vi "Andor_Operate.vi"(8 "error in (no error)":errorcluster, 10 "AndorMainQ":refnum<queue>, 11 "AndorOpQ":refnum<queue>) -> (0 "error out":errorcluster)   [LabVIEW 2019]
uses:
  <userlib>/ATSpectrograph/GUI/AndorNoiseCorr.ctl
  <vilib>/Utility/error.llb/DialogType.ctl
  <userlib>/atmcd32d.llb/Error Code Enum typedef.ctl
panel:
  out "avgfac":i32
  out "Thresh":sgl
  out "cosmic filter":bool
  in  "FilterMode":u32
  out "Dll Error Code":u32
  in  "test filter":bool
  in  "#Curves":u32=1 min=1 max=20 step=1
  out "TempErr":bool
  in  "Backgnd Mode":T1
  out "Background":i32[](array[numeric])
  in  "Standalone":bool
  out "Temp °C":i32
  out "Stable":bool
  in  "Setp. °C":i32=-80
  in  "Quit":bool
  out "CalValues":sgl[](array[numeric])
  in  "Gain":i32(ring) caption="Device Name" items=["Gain  1.0(x)", "Gain  1.7(x)"]
  out "Aquiring":bool
  in  "Continuous Acq.":bool
  in  "AcquireImage":bool
  out "Datas":i32[][][](array[numeric])
  out "Acq Time(ms)":u32
  in  "Accumulations":u16=1 min=1 step=1
  in  "Cooler Enable":bool=TRUE
  in  "Int_time(ms)":u32=10 caption="Integration time(ms)"
  out "Connected":bool
  in  "Stop":bool
  in  "Init":bool
  in  "Tab Control":enum32{"Spectre", "Image"}(tab)
  out "Max WL":sgl
  out "Sum":dbl
  out "Max":u32
  out "Delta":i32
  out "Max X Position":i32[](array[numeric])
  out "Spectral Graph":cluster{"CalValues":sgl[], dbl[]}[](graph)
  out "Max Intensity":i32[](array[numeric])
  out "Graph":dbl[][](graph)
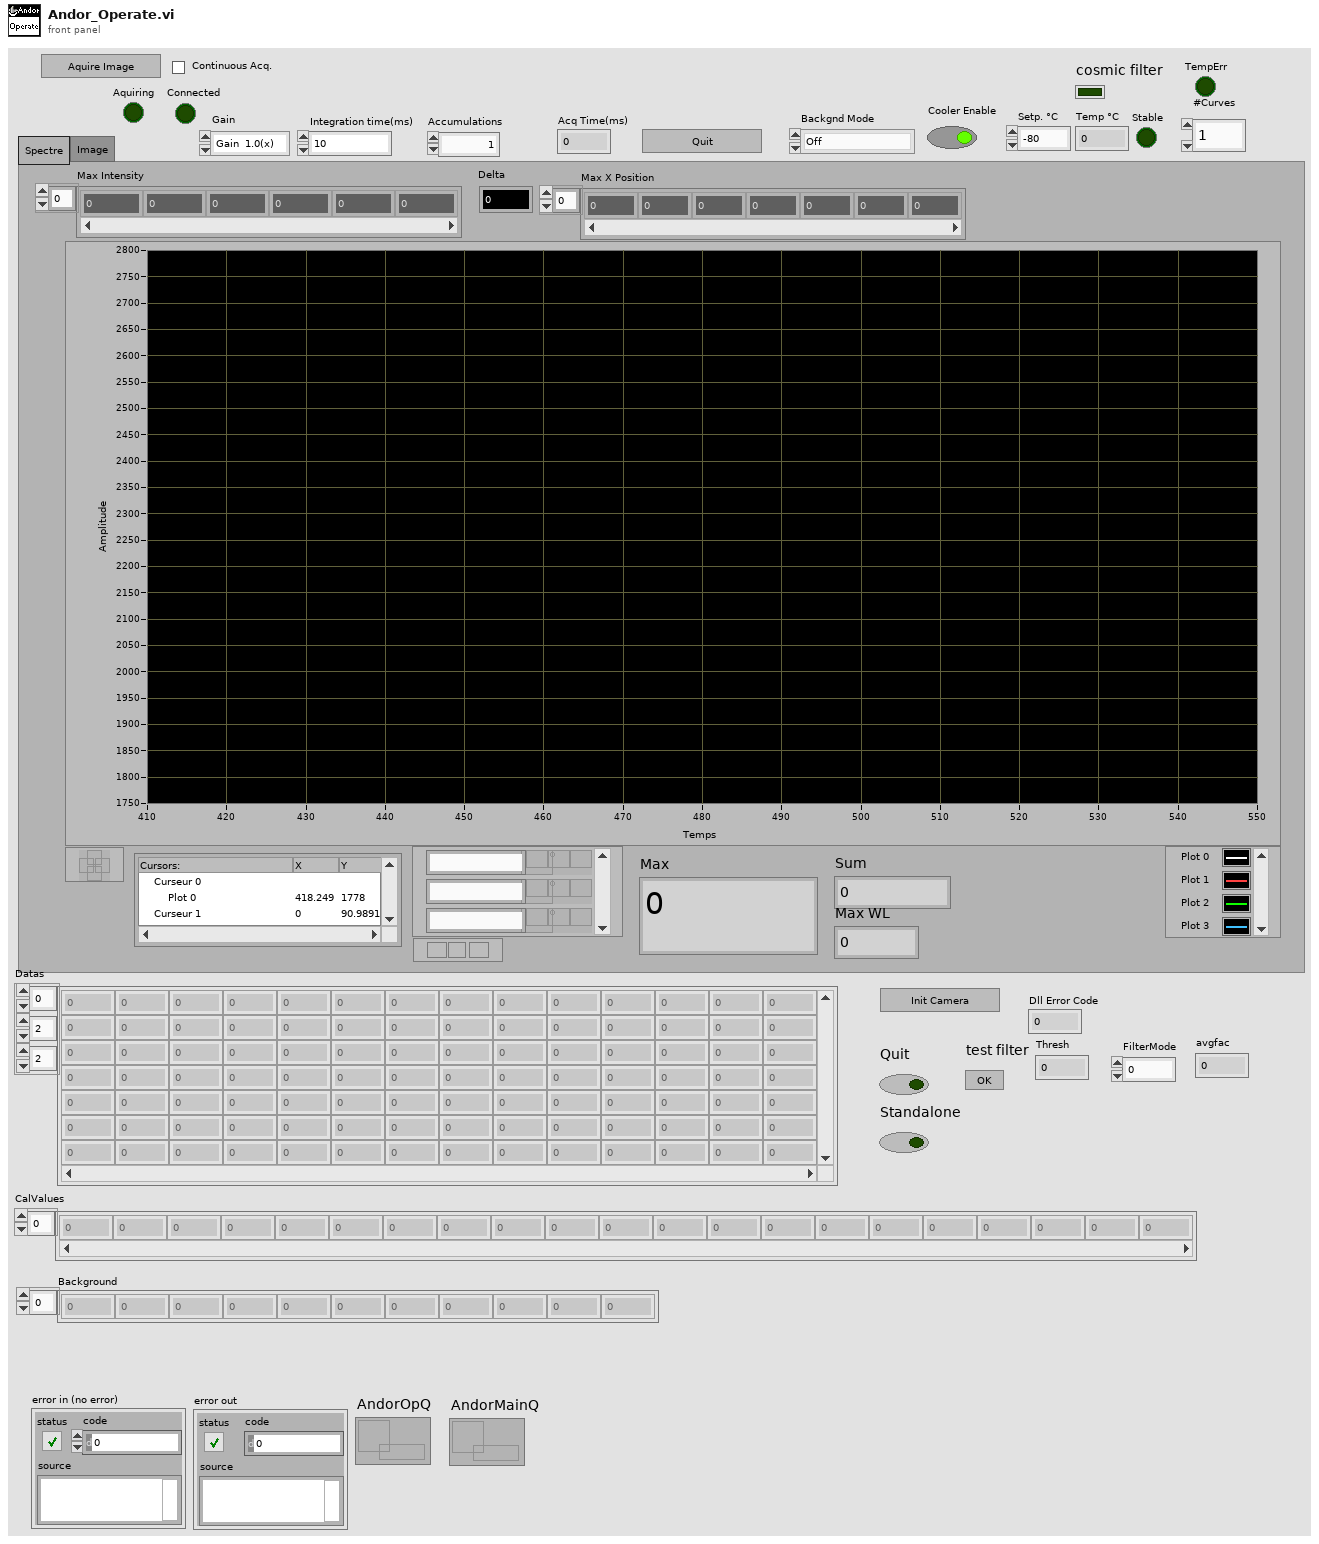
[diagram p1: front panel]
types:
  T1 = typedef "AndorNoiseCorr.ctl" = enum16{"Off", "Selected Curve", "One For Every Acq"}
  T2 = typedef "Error Code Enum typedef.ctl" = enum32{"N/A (0)", "DRV_ERROR_CODES", "DRV_SUCCESS", "DRV_VXDNOTINSTALLED", "DRV_ERROR_SCAN", "DRV_ERROR_CHECK_SUM", "DRV_ERROR_FILELOAD", "DRV_UNKNOWN_FUNC", "DRV_ERROR_VXD_INIT", "DRV_ERROR_ADDRESS", "DRV_ERROR_PAGELOCK", "DRV_ERROR_PAGEUNLOCK", "DRV_ERROR_BOARDTEST", "DRV_ERROR_ACK", "DRV_ERROR_UP_FIFO", "DRV_ERROR_PATTERN", "N/A (16)", "DRV_ACQUISITION_ERRORS", "DRV_ACQ_BUFFER", "DRV_ACQ_DOWNFIFO_FULL", "DRV_PROC_UNKONWN_INSTRUCTION", "DRV_ILLEGAL_OP_CODE", "DRV_KINETIC_TIME_NOT_MET", "DRV_ACCUM_TIME_NOT_MET", "DRV_NO_NEW_DATA", "N/A (25)", "DRV_SPOOLERROR", "N/A (27)", "N/A (28)", "N/A (29)", "N/A (30)", "N/A (31)", "N/A (32)", "DRV_TEMPERATURE_CODES", "DRV_TEMPERATURE_OFF", "DRV_TEMPERATURE_NOT_STABILIZED", "DRV_TEMPERATURE_STABILIZED", "DRV_TEMPERATURE_NOT_REACHED", "DRV_TEMPERATURE_OUT_RANGE", "DRV_TEMPERATURE_NOT_SUPPORTED", "DRV_TEMPERATURE_DRIFT", "N/A (41)", "N/A (42)", "N/A (43)", "N/A (44)", "N/A (45)", "N/A (46)", "N/A (47)", "N/A (48)", "DRV_GENERAL_ERRORS", "DRV_INVALID_AUX", "DRV_COF_NOTLOADED", "DRV_FPGAPROG", "DRV_FLEXERROR", "DRV_GPIBERROR", "N/A (55)", "N/A (56)", "N/A (57)", "N/A (58)", "N/A (59)", "N/A (60)", "N/A (61)", "N/A (62)", "N/A (63)", "DRV_DATATYPE", "DRV_DRIVER_ERRORS", "DRV_P1INVALID", "DRV_P2INVALID", "DRV_P3INVALID", "DRV_P4INVALID", "DRV_INIERROR", "DRV_COFERROR", "DRV_ACQUIRING", "DRV_IDLE", "DRV_TEMPCYCLE", "DRV_NOT_INITIALIZED", "DRV_P5INVALID", "DRV_P6INVALID", "DRV_INVALID_MODE", "DRV_INVALID_FILTER", "DRV_I2CERRORS", "DRV_I2CDEVNOTFOUND", "DRV_I2CTIMEOUT", "DRV_P7INVALID", "N/A (84)", "N/A (85)", "N/A (86)", "N/A (87)", "N/A (88)", "N/A (89)", "DRV_IOCERROR", "DRV_VRMVERSIONERROR"}
  T3 = cluster{"Message":string, "Data":variant, "Code":i32}
  T4 = cluster{"wavelength out":sgl, "calibrationValuesOut":sgl[], "gain":sgl, bool}
  T5 = typedef "DialogType.ctl" = u16
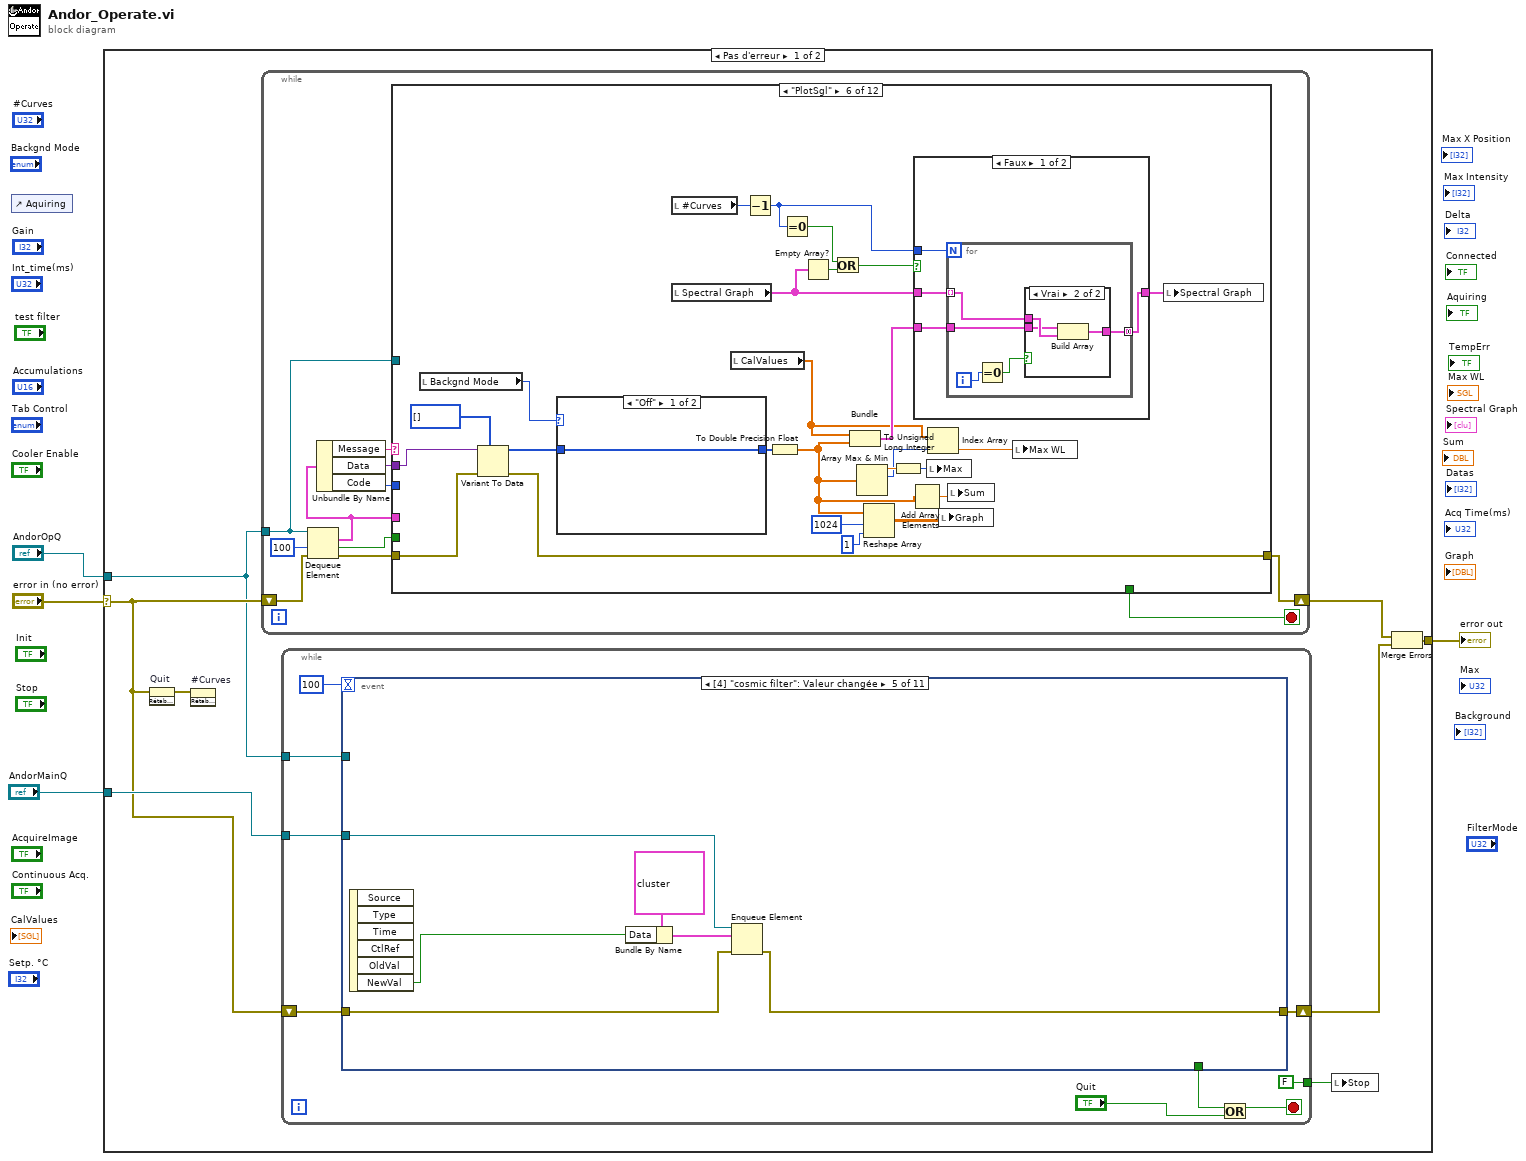
[diagram p0: block diagram]
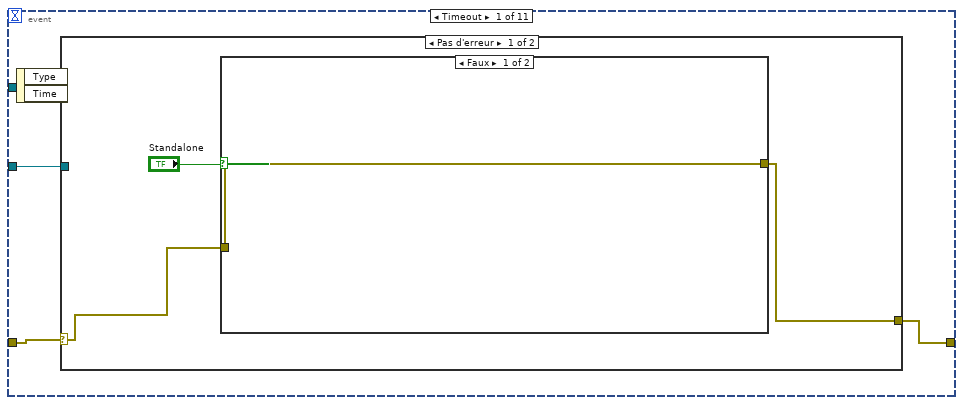
[diagram p2: hidden frame]
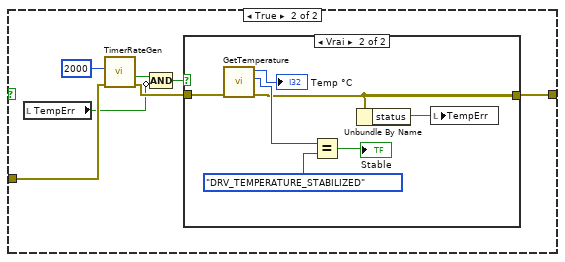
[diagram p3: hidden frame]
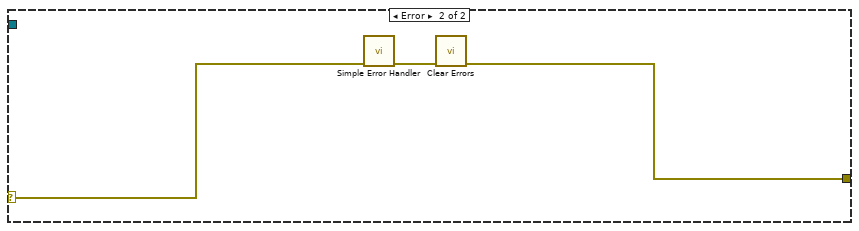
[diagram p5: hidden frame]
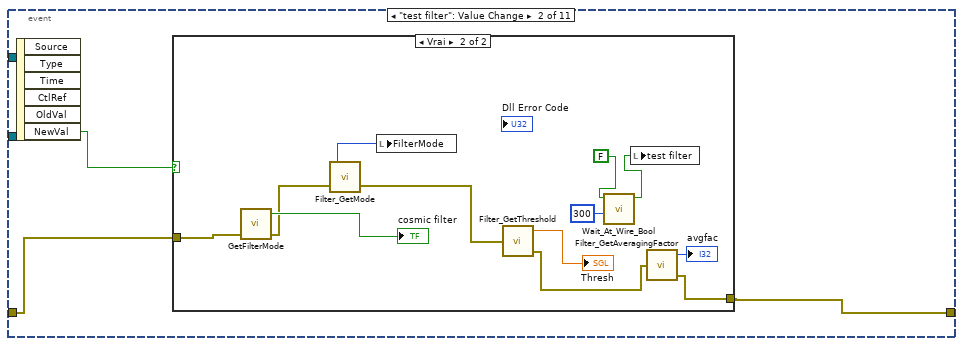
[diagram p6: hidden frame]
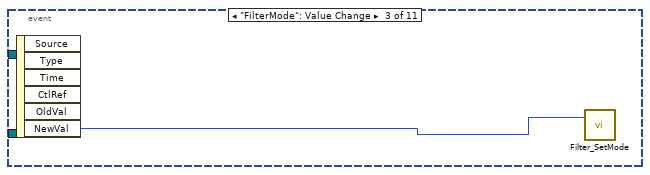
[diagram p8: hidden frame]
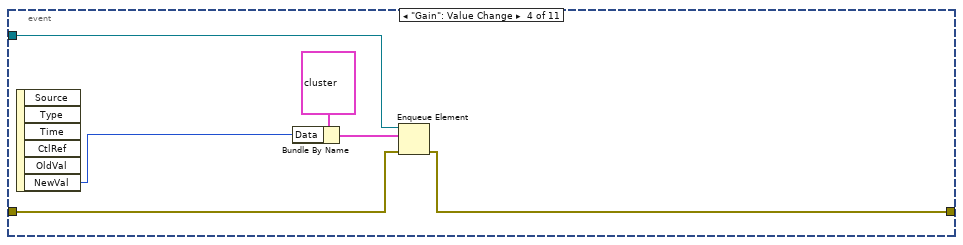
[diagram p9: hidden frame]
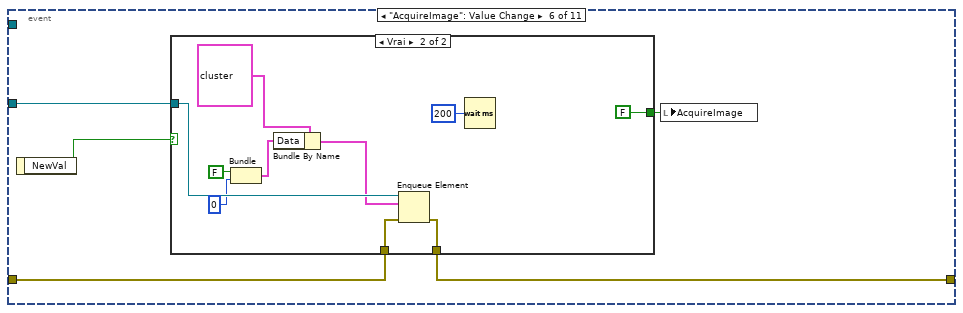
[diagram p10: hidden frame]
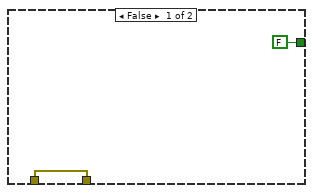
[diagram p11: hidden frame]
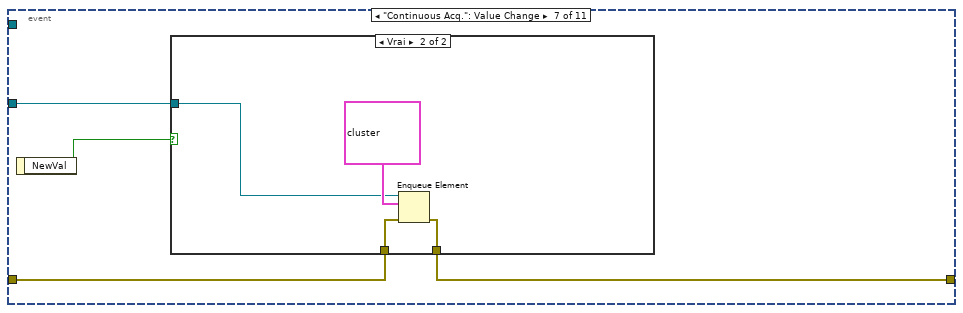
[diagram p12: hidden frame]
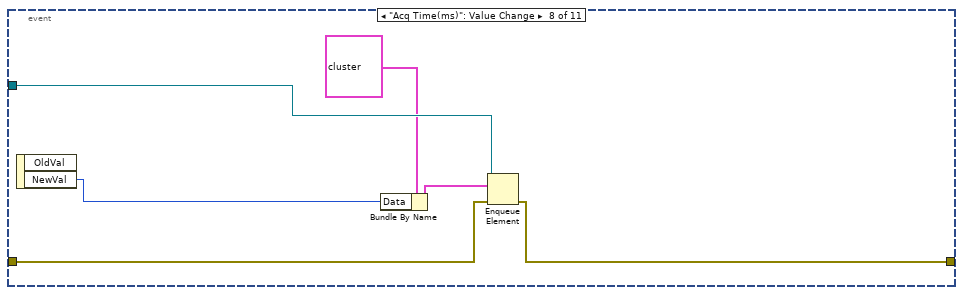
[diagram p14: hidden frame]
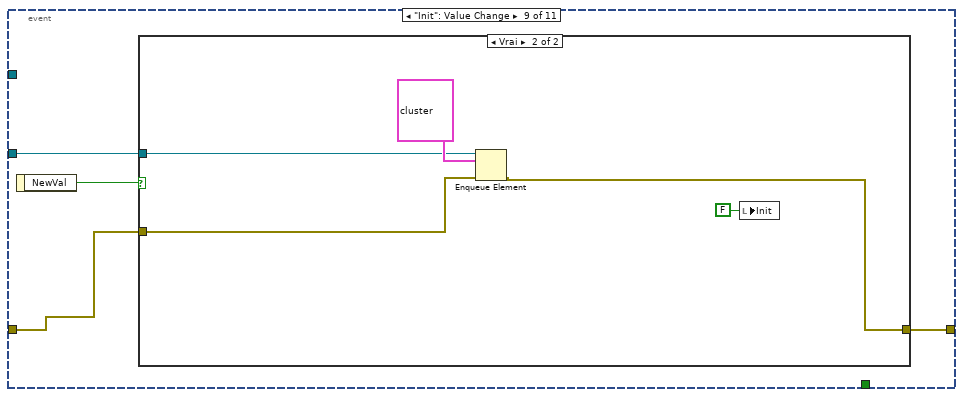
[diagram p15: hidden frame]
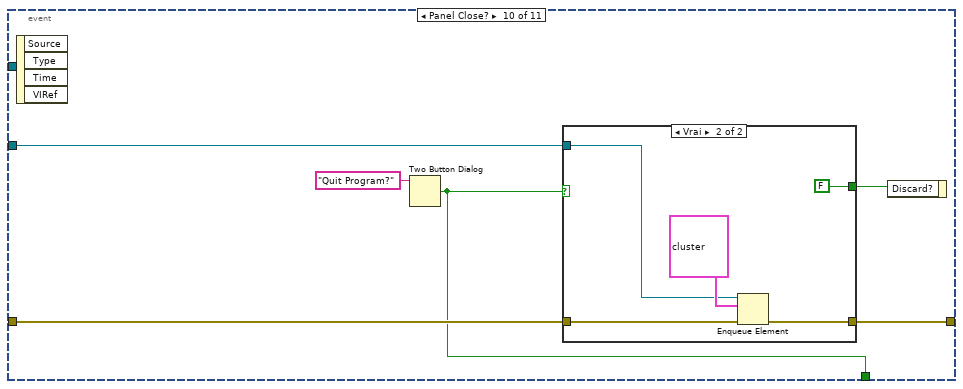
[diagram p17: hidden frame]
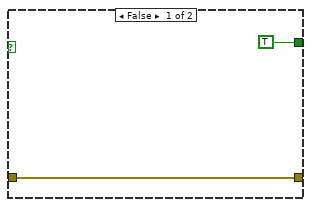
[diagram p18: hidden frame]
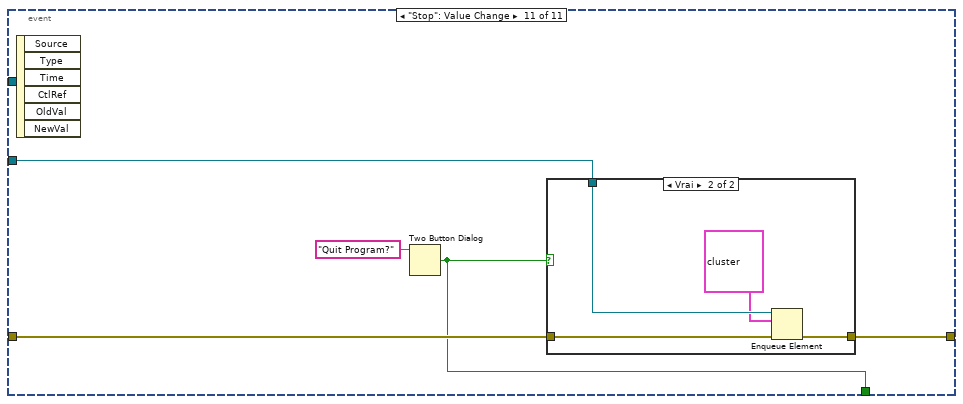
[diagram p19: hidden frame]
diagram:
  n1 = control-ref of="Aquiring"() -> ()  [unwired: 1 out]
  n2 = case shown="Pas d'erreur" "error in (no error)" {
    selector: "error in (no error)" -> [w8 w287]
    tunnel: [w12 w287] -> w3
    tunnel: "AndorMainQ" -> [w10 _]
    tunnel: "AndorOpQ" -> [w7 _]
    frame No Error {
      n3 = invoke on="Quit" class="Bool (strict)" method="RétablirValParDéfaut"(error in=w8) -> (error out=w5:errorcluster)  [unwired: 2 in, 2 out]
      n4 = invoke on="#Curves" class="NumNb (strict)" method="RétablirValParDéfaut"(error in=w5) -> ()  [unwired: 2 in, 3 out]
      n5 = while {
        shift-right: [w141] -> w9
        shift-left: w8 -> [w151]
        tunnel: w7 -> [w145]
        stop <- w148 stop-if-true
        n6 = Dequeue Element(queue=w145, timeout in ms (-1)=100, error in (no error)=w151) -> (element=w146:T3, timed out?=w142:bool, error out=w150:errorcluster)  [unwired: 1 out]
        n7 = Unbundle By Name(w146) -> ("Message"=w149:string, "Data"=w143:variant, "Code"=w144:i32)
        n8 = case shown="\"PlotSgl\"" w149 {
          tunnel: [w152 w158 w164 w191 w196 w223 w254 w262 w268 w274 w279 w284] -> w141
          tunnel: w150 -> [w154 w159 w163 w180 w199 w224 w255 w263 w269 w275 w280 w285]
          tunnel: [w156 FALSE w162 FALSE FALSE _ _ _ _ _ _ _] -> w148
          tunnel: w146 -> [_ _ _ _ _ _ _ _ _ _ _ _]
          tunnel: w145 -> [w155 w160 _ _ _ _ _ _ _ _ _ _]
          tunnel: w144 -> [_ _ _ _ _ _ _ _ _ _ _ _]
          tunnel: w143 -> [_ _ _ w185 w200 w226 w257 w266 w271 w276 w281 w286]
          tunnel: w142 -> [_ _ _ _ _ _ _ _ _ _ _ _]
          frame "Stop" {
            w156 = TRUE
            n9 = Release Queue(queue=w155, error in (no error)=w154) -> (error out=w153:errorcluster)  [unwired: 1 in, 2 out]
            n10 = property on="Quit" class="Bool (strict)"(error in=w153, "Val(Sgnl)"=w156) -> (error out=w152:errorcluster)  [unwired: 1 in, 1 out]
          }
          frame "Standalone" {
            n11 = local write "Standalone"(TRUE ("Standalone")) -> ()
            n12 = Release Queue(queue=w160, error in (no error)=w159) -> (error out=w158:errorcluster)  [unwired: 1 in, 2 out]
          }
          frame "Timeout", Default {
            n13 = Unbundle By Name(w163) -> ("code"=w166:i32)
            n14 = Equal?(x=w166, y=1) -> (x = y?=w162:bool)
            n15 = case shown="Faux" w162 {
              tunnel: [w168 w171] -> w164
              tunnel: w163 -> [w167 w171]
              frame False {
                w170 = T5 1 items=["pas de dialogue", "Message OK", "Message continuer ou arrêter", "Message OK + mises en garde", "Arrêter/Continuer + mises en garde"] ("type of dialog (OK msg:1)")
                n16 = call <vilib>:"General Error Handler.vi"("type of dialog (OK msg:1)"=w170, "error in (no error)"=w167) -> ("error out"=w169:errorcluster)  [unwired: 9 in, 4 out]
                n17 = local write "error out"(w169) -> ()
                n18 = call <vilib>:"Clear Errors.vi"("error in (no error)"=w169) -> ("error out"=w168:errorcluster)  [unwired: 5 in, 1 out]
              }
              frame True {
              }
            }
          }
          frame "InitOp" {
            n19 = invoke on="Connected" class="Bool (strict)" method="RétablirValParDéfaut"(error in=w180) -> (error out=w187:errorcluster)  [unwired: 2 in, 2 out]
            n20 = Reverse 1D Array(array=u32[] [16711680, 16773120, 2359040, 131327, 3080307] ("Sous-tableau")) -> (reversed array=w189:u32[])
            n21 = Variant To Data(error in=w180, type=T4 {"wavelength out"=0.0, "calibrationValuesOut"=[], "gain"=0.0, FALSE} ("cluster"), Variant=w185) -> (data=w183:T4, error out=w182:errorcluster)
            n22 = for {
              tunnel: cluster{dbl, u32}[] [{0.0, 0}, {10923.0, 0}, {21845.0, 0}, {32768.0, 0}, {43691.0, 0}, {54613.0, 0}] ("Z Scale.Marker Values[]") -> [w195] mode=indexing
              tunnel: w189 -> [w194] mode=indexing
              tunnel: [w193] -> w181 mode=indexing
              n23 = Bundle(cluster=w195, w194) -> (w193:cluster{dbl, u32})  [unwired: 1 in]
            }
            n24 = Unbundle By Name(w183) -> ("calibrationValuesOut"=w186:sgl[])  [unwired: 2 out]
            n25 = invoke on="Accumulations" class="NumNb (strict)" method="RétablirValParDéfaut"(error in=w187) -> (error out=w178:errorcluster)  [unwired: 2 in, 2 out]
            n26 = invoke on="Standalone" class="Bool (strict)" method="RétablirValParDéfaut"(error in=w178) -> (error out=w177:errorcluster)  [unwired: 2 in, 2 out]
            n27 = Initialize Array(0, 1024 ("taille de la dimension")) -> (w175:i32[])
            n28 = property on="Graph" class="GraphInt (strict)"(error in=w180, "ZScale.MarkerVals[]"=w181) -> (error out=w179:errorcluster)  [unwired: 1 in, 1 out]
            n29 = local write "CalValues"(w186) -> ()
            n30 = local write "Background"(w175) -> ()
            n31 = invoke on="Backgnd Mode" class="Énum (strict)" method="RétablirValParDéfaut"(error in=w177) -> (error out=w176:errorcluster)  [unwired: 2 in, 2 out]
            n32 = local write "TempErr"(FALSE ("TempErr")) -> ()
            n33 = Merge Errors(w176, w182, w179) -> (w191:errorcluster)
          }
          frame "UpdateWl" {
            n34 = Variant To Data(error in=w199, type=sgl[] [] ("calibrationValuesOut"), Variant=w200) -> (data=w197:sgl[], error out=w196:errorcluster)
            n35 = local write "CalValues"(w197) -> ()
          }
          frame "PlotSgl" {
            n36 = local read "Backgnd Mode"() -> (w217:T1)
            n37 = Variant To Data(error in=w224, type=i32[] [] ("Data out"), Variant=w226) -> (data=w215:i32[], error out=w223:errorcluster)
            n38 = case shown="\"Off\"" w217 {
              tunnel: [w243 w244] -> w216
              tunnel: w215 -> [w243 w246]
              frame "Off" {
              }
              frame "Selected Curve", Default {
                n39 = local read "Background"() -> (w245:i32[])
                n40 = Subtract(x=w246, y=w245) -> (x-y=w244:i32[])
              }
            }
            n41 = local read "#Curves"() -> (w211:u32)
            n42 = local read "Spectral Graph"() -> (w209:cluster{"CalValues":sgl[], dbl[]}[])
            n43 = local read "CalValues"() -> (w203:sgl[])
            n44 = Decrement(x=w211) -> (x-1=w210:u32)
            n45 = To Double Precision Float(number=w216) -> (double precision float=w206:dbl[])
            n46 = Equal To 0?(x=w210) -> (x = 0?=w212:bool)
            n47 = Empty Array?(array=w209) -> (empty?=w213:bool)
            n48 = Or(x=w212, y=w213) -> (x .or. y?=w208:bool)
            n49 = Bundle("CalValues"=w203, w206) -> (w214:cluster{"CalValues":sgl[], dbl[]})  [unwired: 1 in]
            n50 = Array Max & Min(array=w206) -> (max value=w219:dbl, max index (indices)=w204:i32)  [unwired: 2 out]
            n51 = Reshape Array(w206, 1024 ("taille de la dimension"), 1 ("taille de la dimension")) -> (w222:dbl[][])
            n52 = To Unsigned Long Integer(number=w219) -> (unsigned 32bit integer=w218:u32)
            n53 = Add Array Elements(numeric array=w206) -> (sum=w205:dbl)
            n54 = case shown="Faux" w208 {
              tunnel: w214 -> [w230 w242]
              tunnel: w210 -> [w229 _]
              tunnel: w209 -> [w228 _]
              tunnel: [w227 w241] -> w207
              frame False {
                n55 = for {
                  N: w229 -> [_]
                  tunnel: w228 -> [w233] mode=indexing
                  tunnel: w230 -> [w232]
                  tunnel: [w231] -> w227 mode=concatenating
                  i -> [w235]
                  n56 = Equal To 0?(x=w235) -> (x = 0?=w234:bool)
                  n57 = case shown="Vrai" w234 {
                    tunnel: w233 -> [w237 w240]
                    tunnel: w232 -> [_ w239]
                    tunnel: [w236 w238] -> w231
                    frame False {
                      n58 = Build Array(w237) -> (w236:cluster{"CalValues":sgl[], dbl[]}[])
                    }
                    frame True {
                      n59 = Build Array(w239, w240) -> (w238:cluster{"CalValues":sgl[], dbl[]}[])
                    }
                  }
                }
              }
              frame True {
                n60 = Build Array(w242) -> (w241:cluster{"CalValues":sgl[], dbl[]}[])
              }
            }
            n61 = local write "Max"(w218) -> ()
            n62 = Index Array(array=w203, index=w204) -> (element=w202:sgl)
            n63 = local write "Graph"(w222) -> ()
            n64 = local write "Sum"(w205) -> ()
            n65 = local write "Max WL"(w202) -> ()
            n66 = local write "Spectral Graph"(w207) -> ()
          }
          frame "PlotImg" {
            n67 = Variant To Data(error in=w255, type=i32[][] [] ("Data out"), Variant=w257) -> (data=w253:i32[][], error out=w254:errorcluster)
            n68 = local read "CalValues"() -> (w252:sgl[])
            n69 = To Double Precision Float(number=w253) -> (double precision float=w250:dbl[][])
            n70 = Transpose 2D Array(2D array=w250) -> (transposed array=w247:dbl[][])
            n71 = Array Max & Min(array=w247) -> (max value=w249:dbl)  [unwired: 3 out]
            n72 = for {
              tunnel: w250 -> [w260] mode=indexing
              tunnel: w252 -> [w259]
              tunnel: [w258] -> w251 mode=indexing
              n73 = Bundle("CalValues"=w259, w260) -> (w258:cluster{"CalValues":sgl[], dbl[]})  [unwired: 1 in]
            }
            n74 = local write "Graph"(w247) -> ()
            n75 = To Unsigned Long Integer(number=w249) -> (unsigned 32bit integer=w248:u32)
            n76 = local write "Max"(w248) -> ()
            n77 = local write "Spectral Graph"(w251) -> ()
          }
          frame "SetBckGnd" {
            n78 = Variant To Data(error in=w263, type=i32[][] [], Variant=w266) -> (data=w264:i32[][], error out=w262:errorcluster)
            n79 = Index Array(array=w264) -> (element=w261:i32[])  [unwired: 2 in]
            n80 = local write "Background"(w261) -> ()
          }
          frame "SetBckGndMode" {
            n81 = Variant To Data(error in=w269, type=u16 0, Variant=w271) -> (data=w270:u16, error out=w268:errorcluster)
            n82 = local write "Backgnd Mode"(w270) -> ()
          }
          frame "SetInteg" {
            n83 = Variant To Data(error in=w275, type=u32 0, Variant=w276) -> (data=w273:u32, error out=w274:errorcluster)
            n84 = local write "Int_time(ms)"(w273) -> ()
          }
          frame "SetCosmic" {
            n85 = Variant To Data(error in=w280, type=TRUE, Variant=w281) -> (data=w278:bool, error out=w279:errorcluster)
            n86 = local write "cosmic filter"(w278) -> ()
          }
          frame "SetGain" {
            n87 = Variant To Data(error in=w285, type=0, Variant=w286) -> (data=w283:i32, error out=w284:errorcluster)
            n88 = local write "Gain"(w283) -> ()
          }
        }
      }
      n89 = while {
        tunnel: w10 -> [w20]
        shift-right: [w17] -> w11
        shift-left: w8 -> [w18]
        tunnel: w7 -> [w14]
        tunnel: [FALSE ("Stop")] -> w6
        stop <- w16 stop-if-true
        n90 = event shown="[4] \"cosmic filter\": Valeur changée" {
          selector: _ -> [_ _ _ _ _ _ _ _ _ _ _]
          dyn-events: _ -> [_ _ _ _ _ _ _ _ _ _ _]
          timeout: 100 -> [_ _ _ _ _ _ _ _ _ _ _]
          tunnel: w20 -> [w22 _ _ w68 w74 w80 w96 w107 w110 w122 w134]
          tunnel: [_ _ _ _ _ _ _ _ _ w119 w131] -> w19
          tunnel: w18 -> [w23 w48 _ w67 w73 w79 w95 w106 w109 w121 w133]
          tunnel: [w24 w47 _ w66 w72 w78 w94 w105 w108 w120 w132] -> w17
          tunnel: w14 -> [_ _ _ _ _ _ _ _ _ _ _]
          event Timeout {
            n91 = event-data() -> ()  [unwired: 1 in, 2 out]
            n92 = case shown="Pas d'erreur" w23 {
              selector: w23 -> [w26 w44]
              tunnel: [w25 w45] -> w24
              tunnel: w22 -> [_ _]
              frame No Error {
                n93 = case shown="Faux" "Standalone" {
                  tunnel: w26 -> [w28 w34]
                  tunnel: [w28 w31] -> w25
                  frame False {
                  }
                  frame True {
                    n94 = local read "TempErr"() -> (w29:bool)
                    n95 = call <userlib>:"TimerRateGen.vi"("error in (no error)"=w34, "Refresh(ms)"=u32 2000) -> ("error out"=w33:errorcluster, "updated?"=w32:bool)  [unwired: 7 in, 1 out]
                    n96 = Compound Arithmetic op=AND ("Opérateur arithmétique")(w32, invert w29) -> (w30:bool)
                    n97 = case shown="Vrai" w30 {
                      tunnel: w33 -> [w36 w43]
                      tunnel: [w36 w38] -> w31
                      frame False {
                      }
                      frame True {
                        n98 = call <userlib>:"GetTemperature.vi"("error in (no error)"=w43) -> ("error out"=w38:errorcluster, "status"=w40:T2, "temperature"=→"Temp °C":i32)  [unwired: 3 in, 1 out]
                        n99 = Equal?(x=w40, y=Error_Code_Enum_typedef."DRV_TEMPERATURE_STABILIZED" ("status")) -> (x = y?=→"Stable":bool)
                        n100 = Unbundle By Name(w38) -> ("status"=w37:bool)
                        n101 = local write "TempErr"(w37) -> ()
                      }
                    }
                  }
                }
              }
              frame Error {
                n102 = call <vilib>:"Simple Error Handler.vi"("error in (no error)"=w44) -> ("error out"=w46:errorcluster)  [unwired: 4 in, 4 out]
                n103 = call <vilib>:"Clear Errors.vi"("error in (no error)"=w46) -> ("error out"=w45:errorcluster)  [unwired: 5 in, 1 out]
              }
            }
          }
          event "test filter": Value Change {
            n104 = event-data() -> ("NewVal"=w49:bool)  [unwired: 1 in, 5 out]
            n105 = case shown="Vrai" w49 {
              tunnel: w48 -> [w50 w57]
              tunnel: [w50 w52] -> w47
              frame False {
              }
              frame True {
                n106 = call <userlib>:"GetFilterMode.vi"("error in (no error)"=w57) -> ("error out"=w56:errorcluster, "mode"=→"cosmic filter":bool)  [unwired: 2 in, 1 out]
                n107 = call <userlib>:"Filter_GetMode.vi"("error in (no error)"=w56) -> ("error out"=w55:errorcluster, "Mode"=w59:u32)  [unwired: 1 out]
                n108 = local write "FilterMode"(w59) -> ()
                n109 = call <userlib>:"Filter_GetThreshold.vi"("error in (no error)"=w55) -> ("Mode"=→"Thresh":sgl, "error out"=w53:errorcluster)  [unwired: 1 out]
                n110 = call <userlib>:"Wait_At_Wire_Bool.vi"("Wait (ms)"=u32 300, "error in (no error)"=FALSE) -> ("error out"=w61:bool)  [unwired: 7 in, 2 out]
                n111 = local write "test filter"(w61) -> ()
                n112 = call <userlib>:"Filter_GetAveragingFactor.vi"("error in (no error)"=w53) -> ("Mode"=→"avgfac":i32, "error out"=w52:errorcluster)  [unwired: 1 out]
              }
            }
          }
          event "FilterMode": Value Change {
            n113 = event-data() -> ("NewVal"=w63:u32)  [unwired: 1 in, 5 out]
            n114 = call <userlib>:"Filter_SetMode.vi"("Mode"=w63) -> ()  [unwired: 1 in, 2 out]
          }
          event "Gain": Value Change {
            n115 = event-data() -> ("NewVal"=w64:i32)  [unwired: 1 in, 5 out]
            n116 = Bundle By Name(cluster=cluster{"Message":string, "Data":variant, i32} {"Message"="SetGain", "Data"=variant, 0} ("ClassQueue"), "Data"=w64) -> (w65:cluster{"Message":string, "Data":variant, i32})
            n117 = Enqueue Element(queue=w68, element=w65, error in (no error)=w67) -> (error out=w66:errorcluster)  [unwired: 1 in, 2 out]
          }
          event "cosmic filter": Value Change {
            n118 = event-data() -> ("NewVal"=w70:bool)  [unwired: 1 in, 5 out]
            n119 = Bundle By Name(cluster=cluster{"Message":string, "Data":variant, i32} {"Message"="SetCosmic", "Data"=variant, 0} ("ClassQueue"), "Data"=w70) -> (w71:cluster{"Message":string, "Data":variant, i32})
            n120 = Enqueue Element(queue=w74, element=w71, error in (no error)=w73) -> (error out=w72:errorcluster)  [unwired: 1 in, 2 out]
          }
          event "AcquireImage": Value Change {
            n121 = event-data() -> ("NewVal"=w77:bool)  [unwired: 1 in]
            n122 = case shown="Vrai" w77 {
              tunnel: w80 -> [_ w92]
              tunnel: w79 -> [w82 w91]
              tunnel: [w82 w90] -> w78
              tunnel: [FALSE FALSE] -> w76
              frame False {
              }
              frame True {
                n123 = Bundle(FALSE, 0) -> (w84:cluster{bool, i32})  [unwired: 1 in]
                n124 = Bundle By Name(cluster=cluster{"Message":string, "Data":variant, i32} {"Message"="Acquire", "Data"=variant, 0} ("élément"), "Data"=w84) -> (w86:cluster{"Message":string, "Data":variant, i32})
                n125 = Enqueue Element(queue=w92, element=w86, error in (no error)=w91) -> (error out=w90:errorcluster)  [unwired: 1 in, 2 out]
                n126 = Wait (ms)(milliseconds to wait=u32 200) -> ()  [unwired: 1 out]
              }
            }
            n127 = local write "AcquireImage"(w76) -> ()
          }
          event "Continuous Acq.": Value Change {
            n128 = event-data() -> ("NewVal"=w93:bool)  [unwired: 1 in]
            n129 = case shown="Vrai" w93 {
              tunnel: w96 -> [_ w100]
              tunnel: w95 -> [w97 w99]
              tunnel: [w97 w98] -> w94
              frame False {
              }
              frame True {
                n130 = Enqueue Element(queue=w100, element=cluster{"Message":string, "Data":variant, i32} {"Message"="AcquireLive", "Data"=variant, 0} ("ClassQueue"), error in (no error)=w99) -> (error out=w98:errorcluster)  [unwired: 1 in, 2 out]
              }
            }
          }
          event "Acq Time(ms)": Value Change {
            n131 = event-data() -> ("NewVal"=w104:u32)  [unwired: 1 in, 1 out]
            n132 = Bundle By Name(cluster=T3 {"Message"="SetInteg", "Data"=variant, "Code"=1}, "Data"=w104) -> (w103:T3)
            n133 = Enqueue Element(queue=w107, element=w103, error in (no error)=w106) -> (error out=w105:errorcluster)  [unwired: 1 in, 2 out]
          }
          event "Init": Value Change {
            n134 = event-data() -> ("NewVal"=w111:bool)  [unwired: 1 in]
            n135 = case shown="Vrai" w111 {
              tunnel: w110 -> [_ w113]
              tunnel: w109 -> [w112 w114]
              tunnel: [w112 w115] -> w108
              frame False {
              }
              frame True {
                n136 = Enqueue Element(queue=w113, element=T3 {"Message"="InitCam", "Data"=variant, "Code"=0}, error in (no error)=w114) -> (error out=w115:errorcluster)  [unwired: 1 in, 2 out]
                n137 = local write "Init"(FALSE ("Init")) -> ()
              }
            }
          }
          event Panel Close? {
            n138 = event-data() -> ()  [unwired: 1 in, 4 out]
            n139 = Two Button Dialog(message="Quit Program?") -> (T button?=w119:bool)  [unwired: 2 in]
            n140 = case shown="Vrai" w119 {
              tunnel: w122 -> [_ w129]
              tunnel: w121 -> [w125 w128]
              tunnel: [w125 w127] -> w120
              tunnel: [TRUE FALSE ("Stop")] -> w118
              frame False {
              }
              frame True {
                n141 = Enqueue Element(queue=w129, element=cluster{"Message":string, "Data":variant, i32} {"Message"="CloseOp", "Data"=variant, 0}, error in (no error)=w128) -> (error out=w127:errorcluster)  [unwired: 1 in, 2 out]
              }
            }
            n142 = event-data("Discard?"=w118) -> ()  [unwired: 1 in, 1 out]
          }
          event "Stop": Value Change {
            n143 = event-data() -> ()  [unwired: 1 in, 6 out]
            n144 = Two Button Dialog(message="Quit Program?") -> (T button?=w131:bool)  [unwired: 2 in]
            n145 = case shown="Vrai" w131 {
              tunnel: w134 -> [_ w140]
              tunnel: w133 -> [w136 w139]
              tunnel: [w136 w137] -> w132
              frame False {
              }
              frame True {
                n146 = Enqueue Element(queue=w140, element=cluster{"Message":string, "Data":variant, i32} {"Message"="CloseOp", "Data"=variant, 0}, error in (no error)=w139) -> (error out=w137:errorcluster)  [unwired: 1 in, 2 out]
              }
            }
          }
        }
        n147 = Or(x=w19, y="Quit") -> (x .or. y?=w16:bool)
      }
      n148 = local write "Stop"(w6) -> ()
      n149 = Merge Errors(w9, w11) -> (w12:errorcluster)
    }
    frame Error {
    }
  }
  "error out" <- w3
